vi "Control.vi"() -> ()   [LabVIEW 2025]
panel:
  in  "40":bool
  in  "70":bool
  in  "100":bool
  in  "Don't moove":bool
  in  "L":bool
  in  "D":bool
  in  "R":bool
  in  "U":bool
  in  "stop":bool
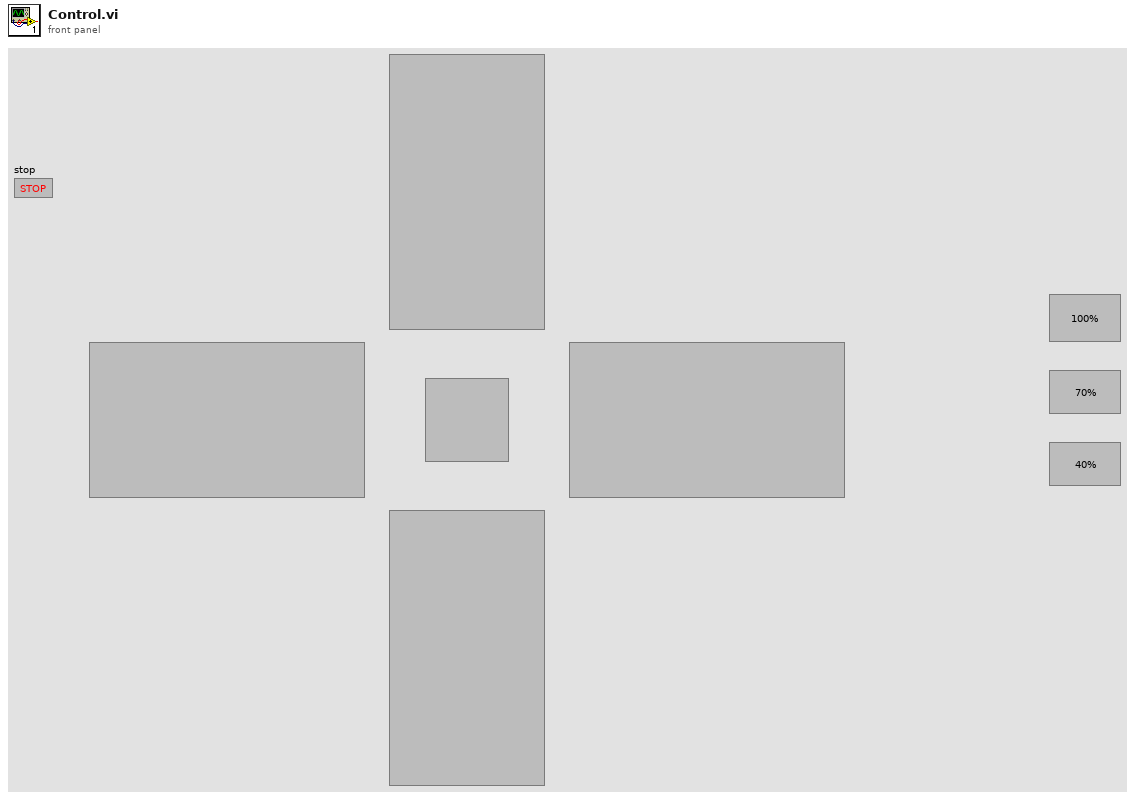
[diagram p1: front panel]
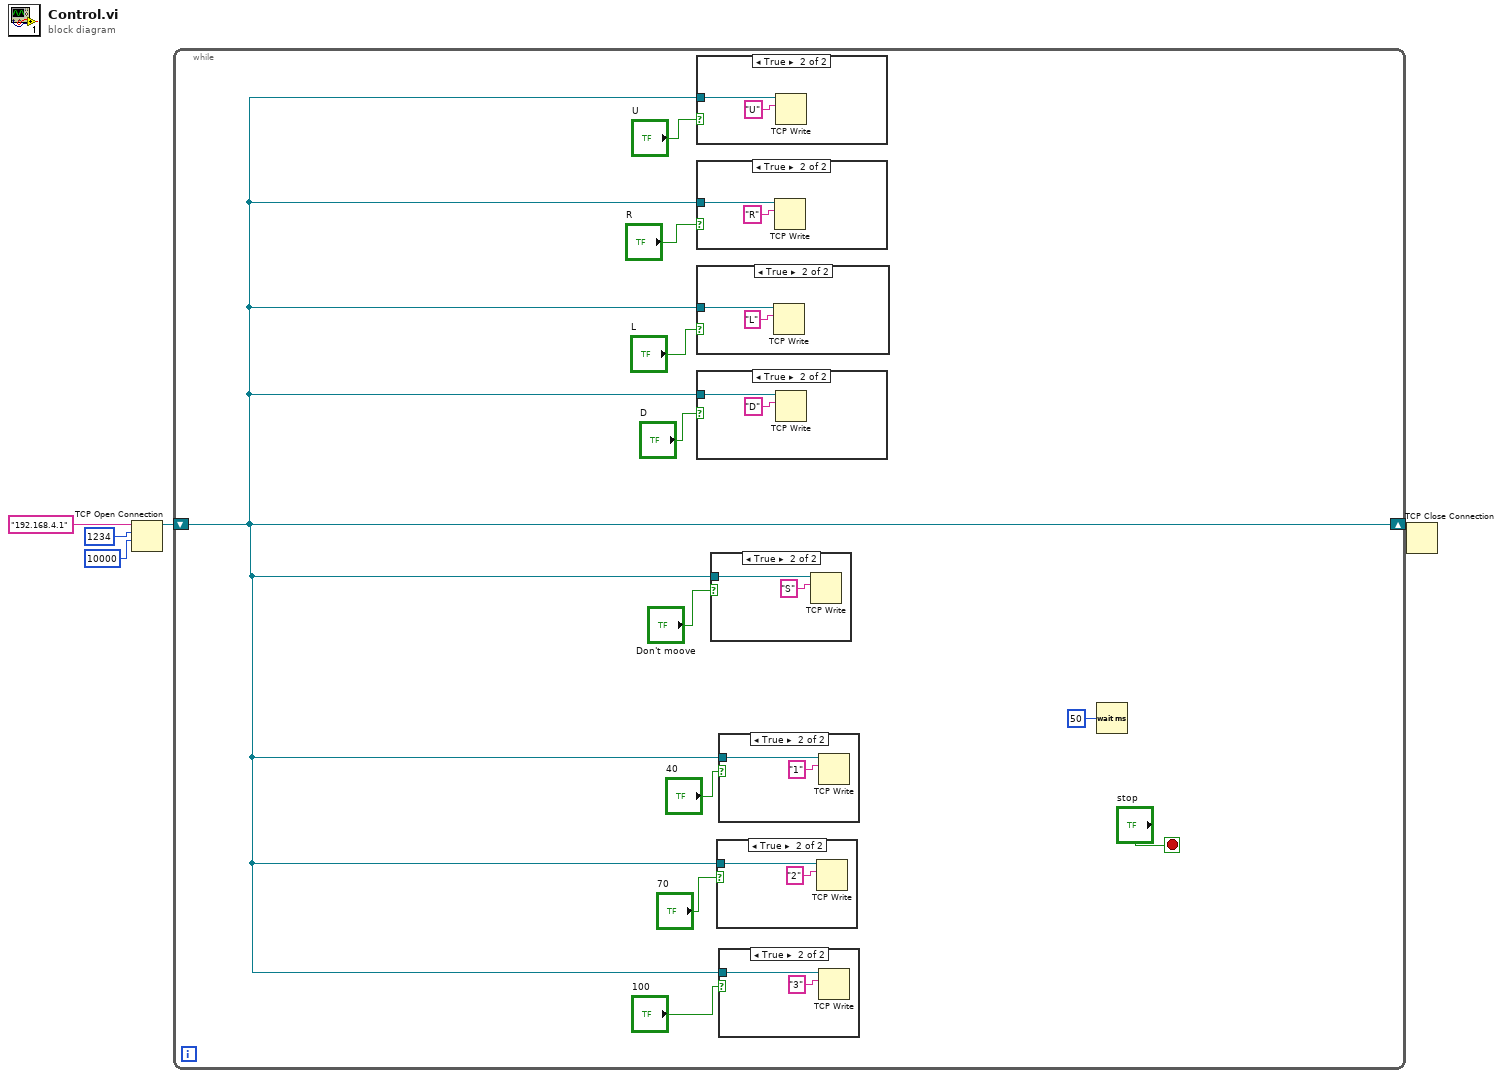
[diagram p0: block diagram]
diagram:
  n1 = TCP Open Connection(address="192.168.4.1", remote port or service name=u16 1234, timeout ms (60000)=10000) -> (connection ID=w3:refnum<k5>)  [unwired: 2 in, 1 out]
  n2 = while {
    shift-right: [w6] -> w2
    shift-left: w3 -> [w6]
    stop <- "stop" stop-if-true
    n3 = case shown="True" "U" {
      tunnel: w6 -> [_ w32]
      frame False {
      }
      frame True {
        n4 = TCP Write(connection ID=w32, data in="U") -> ()  [unwired: 2 in, 3 out]
      }
    }
    n5 = case shown="True" "R" {
      tunnel: w6 -> [_ w30]
      frame False {
      }
      frame True {
        n6 = TCP Write(connection ID=w30, data in="R") -> ()  [unwired: 2 in, 3 out]
      }
    }
    n7 = case shown="True" "L" {
      tunnel: w6 -> [_ w26]
      frame False {
      }
      frame True {
        n8 = TCP Write(connection ID=w26, data in="L") -> ()  [unwired: 2 in, 3 out]
      }
    }
    n9 = case shown="True" "D" {
      tunnel: w6 -> [_ w28]
      frame False {
      }
      frame True {
        n10 = TCP Write(connection ID=w28, data in="D") -> ()  [unwired: 2 in, 3 out]
      }
    }
    n11 = case shown="True" "Don't moove" {
      tunnel: w6 -> [_ w24]
      frame False {
      }
      frame True {
        n12 = TCP Write(connection ID=w24, data in="S") -> ()  [unwired: 2 in, 3 out]
      }
    }
    n13 = case shown="True" "70" {
      tunnel: w6 -> [_ w20]
      frame False {
      }
      frame True {
        n14 = TCP Write(connection ID=w20, data in="2") -> ()  [unwired: 2 in, 3 out]
      }
    }
    n15 = case shown="True" "40" {
      tunnel: w6 -> [_ w22]
      frame False {
      }
      frame True {
        n16 = TCP Write(connection ID=w22, data in="1") -> ()  [unwired: 2 in, 3 out]
      }
    }
    n17 = case shown="True" "100" {
      tunnel: w6 -> [_ w18]
      frame False {
      }
      frame True {
        n18 = TCP Write(connection ID=w18, data in="3") -> ()  [unwired: 2 in, 3 out]
      }
    }
    n19 = Wait (ms)(milliseconds to wait=u32 50) -> ()  [unwired: 1 out]
  }
  n20 = TCP Close Connection(connection ID=w2) -> ()  [unwired: 2 in, 2 out]
